vi "Send Notification Msg.vi"(8 "error in (no error)":errorcluster, 9 "Publication Time (Use Current Time)":timestamp, 10 "Value":variant, 11 "Notification Msg in":refnum<class "Notification Msg.lvclass">) -> (0 "error out":errorcluster)   [LabVIEW 2017, in "Transport.lvlib" / "Notification Msg.lvclass"]
doc: "<License>\nCopyright © 2017 Composed Systems, LLC | All rights reserved\nwww.composed.io\n\nAuthor: Ethan Stern <ethan.stern@composed.io>\n\nThis software is provided \"AS IS\" WITHOUT WARRANTIES, either express or implied, AND IS FOR EDUCATIONAL PURPOSES ONLY.\n</License>"
uses:
  Notification Msg.lvclass
  C:/Git/mva-framework/Framework/AbstractMessages/PreAddressedMsg/PreAddressedMsg.lvclass
  C:/Program Files (x86)/National Instruments/LabVIEW 2017/vi.lib/ActorFramework/Message/Message.lvclass
  AbstractMessages/PreAddressedMsg/PreAddressedMsg.lvclass/PreAddressedMsg.ctl
  Notification Msg.lvclass/Notification Msg.ctl
  <vilib>/ActorFramework/Message Enqueuer/Message Enqueuer.lvclass/Message Enqueuer.ctl
  <vilib>/ActorFramework/Message Priority Queue/Priority Enqueue.vi
  <vilib>/ActorFramework/Message Enqueuer/Message Enqueuer.lvclass
  AbstractMessages/PreAddressedMsg/PreAddressedMsg.lvclass
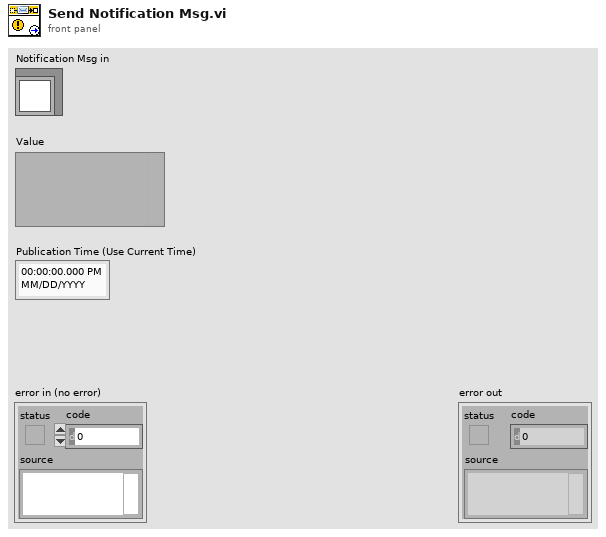
[diagram p1: front panel]
types:
  T1 = typedef "Actor Framework.lvlib/Message Enqueuer.lvclass/Message Priority.ctl" = enum16{"Low", "Normal", "High"}
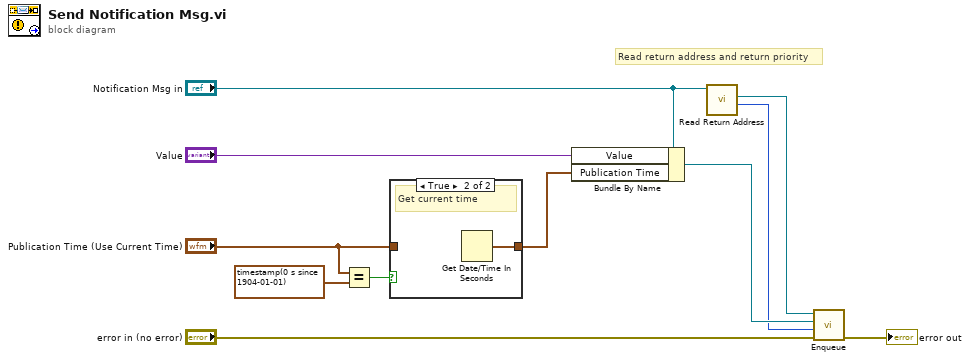
[diagram p0: block diagram]
diagram:
  # "Read return address and return priority"
  n1 = Equal?(x="Publication Time (Use Current Time)", y=timestamp(0 s since 1904-01-01)) -> (x = y?=w3:bool)
  n2 = case shown="True" w3 {
    tunnel: "Publication Time (Use Current Time)" -> [w12 _]
    tunnel: [w12 w13] -> w1
    frame False {
      # "Use input time"
    }
    frame True {
      # "Get current time"
      n3 = Get Date/Time In Seconds() -> (seconds since 1Jan1904=w13:timestamp)
    }
  }
  n4 = Bundle By Name(cluster="Notification Msg in", "Value"="Value", "Publication Time"=w1) -> (w6:refnum<class "Notification Msg.lvclass">)
  n5 = call "Read Return Address.vi"("PreAddressedMsg in"="Notification Msg in") -> ("Return Priority (Normal)"=w5:T1, "Return Address"=w7:refnum<class "Message Enqueuer.lvclass">)  [unwired: 9 in]
  n6 = call <vilib>:"Enqueue.vi"("error in (no error)"="error in (no error)", "Message Priority (Normal)"=w5, "Message"=w6, "Message Enqueuer in"=w7) -> ("error out"=→"error out":errorcluster)  [unwired: 6 in, 1 out]
